vi "Wrapper_getSpectrum.vi"(2 "Index":i32, 3 "Wrapper":u32) -> (0 "Length":i32, 1 "Spectrum Values":dbl[](array[numeric]))   [LabVIEW 2012]
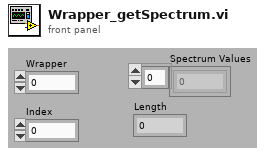
[diagram p1: front panel]
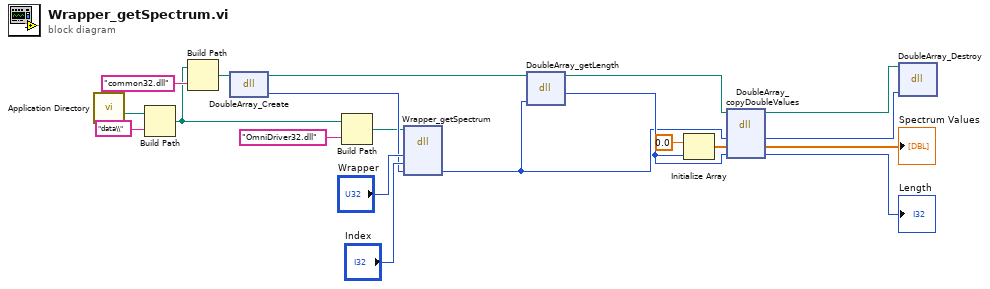
[diagram p0: block diagram]
diagram:
  n1 = call <vilib>:"Application Directory.vi"() -> ("Application Directory"=w7:path)
  n2 = Build Path(base path=w7, name or relative path="data\\") -> (appended path=w3:path)
  n3 = Build Path(base path=w3, name or relative path="common32.dll") -> (appended path=w2:path)
  n4 = dll-call lib="common32.dll" fn="DoubleArray_Create" label="DoubleArray.Create"(path in=w2) -> (path out=w8:path, "return type"=w18:u32)  [unwired: 2 in, 1 out]
  n5 = Build Path(base path=w3, name or relative path="OmniDriver32.dll") -> (appended path=w1:path)
  n6 = dll-call lib="D:/Software Development/EPI Development/BurnIn Testing/Instruments/Drivers/Ocean Optics/OOI_HOME/OmniDriver32.dll" fn="Wrapper_getSpectrum" label="Wrapper.getSpectrum"(path in=w1, "Wrapper"="Wrapper", "Index"="Index", "DoubbleArray"=w18) -> ("DoubbleArray"=w14:u32)  [unwired: 4 in, 3 out]
  n7 = dll-call lib="common32.dll" fn="DoubleArray_getLength" label="DoubleArray.getLength"(path in=w8, "DoubbleArray"=w14) -> (path out=w9:path, "return type"=w15:i32)  [unwired: 3 in, 1 out]
  n8 = Initialize Array(0.0 ("element"), w15) -> (w16:dbl[])
  n9 = dll-call lib="common32.dll" fn="DoubleArray_copyDoubleValues" label="DoubleArray.copyDoubleValues"(path in=w9, "DoubbleArray"=w14, "Values"=w16, "Length"=w15) -> (path out=w10:path, "DoubbleArray"=w11:u32, "Values"=→"Spectrum Values":dbl[], "Length"=→"Length":i32)  [unwired: 2 in, 2 out]
  n10 = dll-call lib="common32.dll" fn="DoubleArray_Destroy" label="DoubleArray.Destroy"(path in=w10, "DoubleArray"=w11) -> ()  [unwired: 3 in, 3 out]
